vi "删除2D数组元素(DBL).vi"(8 "error in (no error)":errorcluster caption="错误输入（无错误）", 9 "选择行列":enum16{"行", "列"}(ring), 10 "索引":i32[](array[numeric]), 11 "输入数组":dbl[][](array[numeric])) -> (0 "error out":errorcluster caption="错误输出", 2 "已删除元素":dbl[][](array[numeric]) format="%.2f", 3 "剩余元素":dbl[][](array[numeric]) format="%.2f")   [LabVIEW 2011]
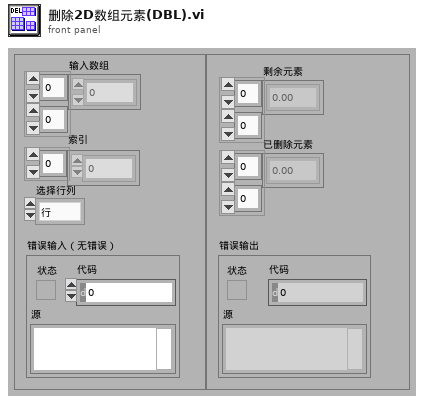
[diagram p1: front panel]
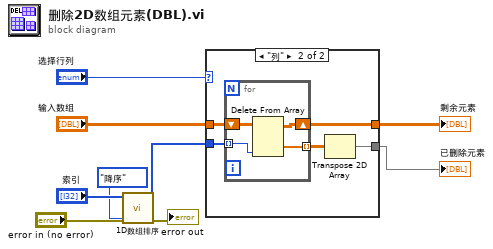
[diagram p0: block diagram]
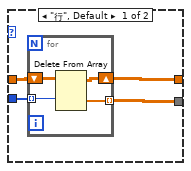
[diagram p2: hidden frame]
diagram:
  n1 = call-poly "1D数组排序.vi"("error in (no error)"="error in (no error)", "升降序"=enum16{"升序", "降序"}."降序", "输入数组"="索引") -> ("error out"=→"error out":errorcluster, "排序后数组"=w3:i32[])  [unwired: 6 in, 1 out]
  n2 = case shown="\"列\"" "选择行列" {
    tunnel: "输入数组" -> [w13 w22]
    tunnel: w3 -> [w12 w21]
    tunnel: [w11 w18] -> w4
    tunnel: [w10 w19] -> w1
    frame "行", Default {
      n3 = for {
        shift-right: [w15] -> w11
        shift-left: w13 -> [w17]
        tunnel: w12 -> [w16] mode=indexing
        tunnel: [w14] -> w10 mode=indexing
        n4 = Delete From Array(array=w17, index (row)=w16) -> (deleted portion=w14:dbl[], array with subset deleted=w15:dbl[][])  [unwired: 2 in]
      }
    }
    frame "列" {
      n5 = for {
        shift-right: [w24] -> w18
        shift-left: w22 -> [w26]
        tunnel: w21 -> [w25] mode=indexing
        tunnel: [w23] -> w20 mode=indexing
        n6 = Delete From Array(array=w26, index (col)=w25) -> (deleted portion=w23:dbl[], array with subset deleted=w24:dbl[][])  [unwired: 2 in]
      }
      n7 = Transpose 2D Array(2D array=w20) -> (transposed array=w19:dbl[][])
    }
  }
  "剩余元素" <- w4
  "已删除元素" <- w1
